vi "Message - Acknowledge.vi"(0 "Message In":string="MESSAGE", 3 "error in":errorcluster) -> (10 "error out":errorcluster)   [LabVIEW 2014]
panel:
  out "Message Out":string="MESSAGE"
  in  "Acknowledge Button":bool
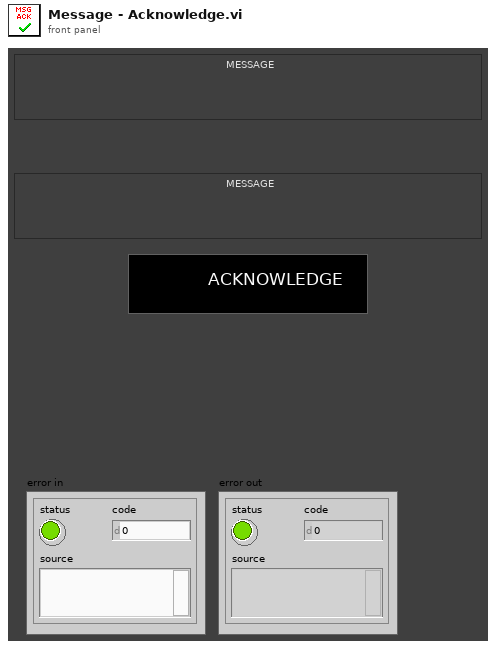
[diagram p1: front panel]
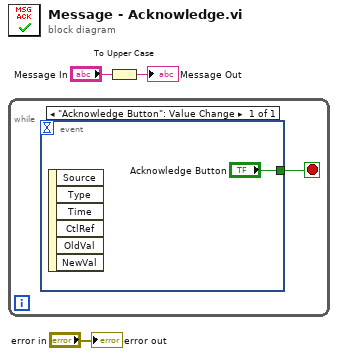
[diagram p0: block diagram]
diagram:
  n1 = while {
    stop <- w4 stop-if-true
    n2 = event shown="[0] \"Acknowledge Button\": Value Change" {
      selector: _ -> [_]
      dyn-events: _ -> [_]
      timeout: _ -> [_]
      tunnel: ["Acknowledge Button"] -> w4
      event "Acknowledge Button": Value Change {
        n3 = event-data() -> ()  [unwired: 1 in, 6 out]
      }
    }
  }
  n4 = To Upper Case(1:"Message In") -> (0:→"Message Out":string)
  "error out" <- "error in"
